vi "Test ADC Rate (Session).vi"() -> ()   [LabVIEW 2020, in "CTI-Scratchpad.lvlib"]
uses:
  CTI-Scratchpad.lvlib
  CTI/Error Reporting.ctl
  CTI/ADC Number.ctl
  CTI/Session/Session.lvclass
  <vilib>/ptbypt/NI_PtbyPt.lvlib
  CTI/VisaComms/VisaComms.lvclass
  CTI/CTI.lvlib
panel:
  in  "Error Checking (Full)":T1=enum."Full"
  in  "stop":bool
  out "ADC":dbl[][](graph)=[[2063.0, 0.0007534999895142391, 756.5504025676244]]
  in  "Port":refnum<visa-resource-name>="COM3"
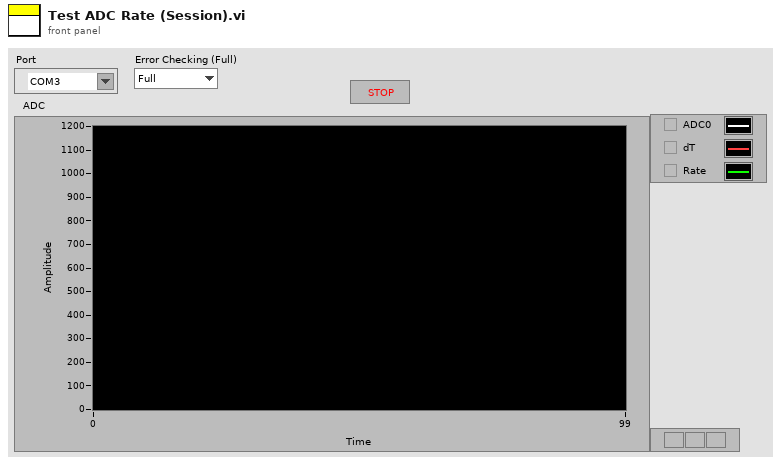
[diagram p1: front panel]
types:
  T1 = typedef "CTI.lvlib/Error Reporting.ctl" = enum16{"Minimal", "Moderate", "Full"}
  T2 = typedef "CTI.lvlib/ADC Number.ctl" = i8
  T3 = typedef "CTI.lvlib/Raw ADC.ctl" = u16
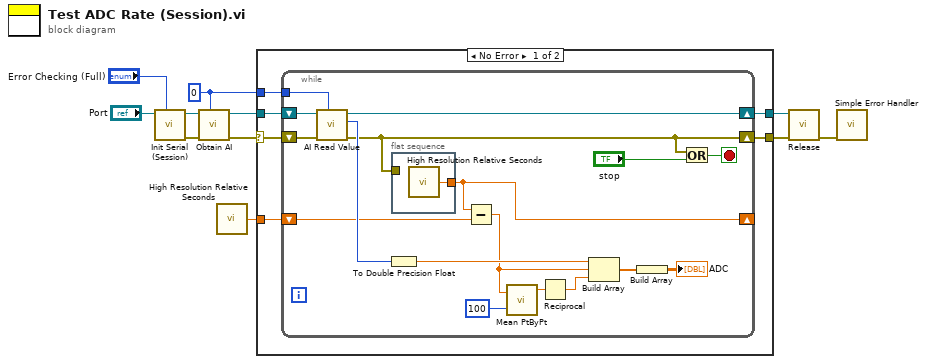
[diagram p0: block diagram]
diagram:
  w2 = T2 0 ("Channel")
  n1 = call "Init Serial (Session).vi"("Error Checking (Full)"="Error Checking (Full)", "VISA resource name in"="Port") -> ("error out"=w9:errorcluster, "Session"=w10:refnum<class "Session.lvclass">)  [unwired: 7 in, 1 out]
  n2 = call "Obtain AI.vi"("ADC #"=w2, "error in (no error)"=w9, "Session in"=w10) -> ("error out"=w8:errorcluster, "Session out"=w3:refnum<class "Session.lvclass">)  [unwired: 7 in]
  n3 = call <vilib>:"High Resolution Relative Seconds.vi"() -> ("relative seconds"=w4:dbl)
  n4 = case shown="No Error" w8 {
    selector: w8 -> [w15 w37]
    tunnel: w3 -> [w16 w36]
    tunnel: w2 -> [w17 _]
    tunnel: [w13 w37] -> w6
    tunnel: [w14 w36] -> w7
    tunnel: w4 -> [w12 _]
    frame No Error {
      n5 = while {
        tunnel: w17 -> [w18]
        shift-right: [w32] -> w14
        shift-left: w16 -> [w34]
        shift-right: [w28] -> w13
        shift-left: w15 -> [w33]
        shift-right: [w25] -> _
        shift-left: w12 -> [w26]
        stop <- w31 stop-if-true
        n6 = call "AI Read Value.vi"("ADC #"=w18, "error in (no error)"=w33, "Session in"=w34) -> ("error out"=w28:errorcluster, "Value"=w30:T3, "Session out"=w32:refnum<class "Session.lvclass">)  [unwired: 6 in]
        n7 = To Double Precision Float(number=w30) -> (double precision float=w24:dbl)
        n8 = flat-sequence {
          tunnel: w28 -> [_]
          tunnel: [w35] -> w25
          frame #0 {
            n9 = call <vilib>:"High Resolution Relative Seconds.vi"() -> ("relative seconds"=w35:dbl)
          }
        }
        n10 = Subtract(x=w25, y=w26) -> (x-y=w23:dbl)
        n11 = call <vilib>:"Mean PtByPt.vi"("x"=w23, "sample length"=100) -> ("mean"=w21:dbl)  [unwired: 2 in, 1 out]
        n12 = Reciprocal(x=w21) -> (1/x=w20:dbl)
        n13 = Build Array(w24, w23, w20) -> (w29:dbl[])
        n14 = Build Array(w29) -> (→"ADC":dbl[][])
        n15 = Or(x=w28, y="stop") -> (x .or. y?=w31:bool)
      }
    }
    frame Error {
    }
  }
  n16 = call-dynamic "Release.vi"("error in (no error)"=w6, "Session in"=w7) -> ("error out"=w5:errorcluster)  [unwired: 9 in]
  n17 = call <vilib>:"Simple Error Handler.vi"("error in (no error)"=w5) -> ()  [unwired: 4 in, 5 out]
